vi "SelectMenu3.vi"(6 "Click Type":T1, 7 "Id":string, 8 "Point":T8, 9 "Item Index":u32, 10 "XRef":refnum<vi>, 11 "State In":T2={"Input Type"=variant(dbl 0.0), "Width"=0, "Typedef Name"="", "Value Type"=variant, "Selection"=0, "Options"=[], "Selections"=[], "Display Selections"=[], "Element Names"=[], "Typedef Name Width"=0, "Display Selection Width"=[], "Code Generated"=FALSE}) -> (0 "Reply":string[](array[string]), 3 "State Out":T2={"Input Type"=variant(dbl 0.0), "Width"=0, "Typedef Name"="", "Value Type"=variant, "Selection"=0, "Options"=[], "Selections"=[], "Display Selections"=[], "Element Names"=[], "Typedef Name Width"=0, "Display Selection Width"=[], "Code Generated"=FALSE})   [LabVIEW 2015, in "Read-Write-Signals.xnode"]
doc: "This ability VI is called after the user selects an item from a portion of the menu defined during BuildMenu. Click Type is the type of click that led to the building of the menu whose selection is being handled by this VI. ItemIndex is the index of the element in the array used when you specified the popup menu. Id is the id you associated with the item in BuildMenu3. Point is the location where the user clicked to build the menu relative to the top-left corner of the XNode. You can display a dialog in response to a user selection if you wish. Use Reply to inform LabVIEW of any actions it needs to take.\n\nDefault behavior: None.\n\nThis ability provides UI and OS messages are handled.\n\nSee also: BuildMenu3"
uses:
  Read-Write-Signals.xnode
  State.ctl
  Read-Write-Signals Item.ctl
  Read-Write-Signals Sub Item.ctl
  Read-Write-Signals Sub Item Type.ctl
  Read-Write-Signals Selection.ctl
  Read-Write-Signals Display Selection.ctl
  <vilib>/XNodeSupport/XNodePoint.ctl
  <vilib>/XNodeSupport/XNodeInt.ctl
  <vilib>/XNodeSupport/XNodeClickTypes.ctl
  <vilib>/regexp/Match Regular Expression.xnode
  <vilib>/XNodeSupport/NI_XNodeSupport.lvlib
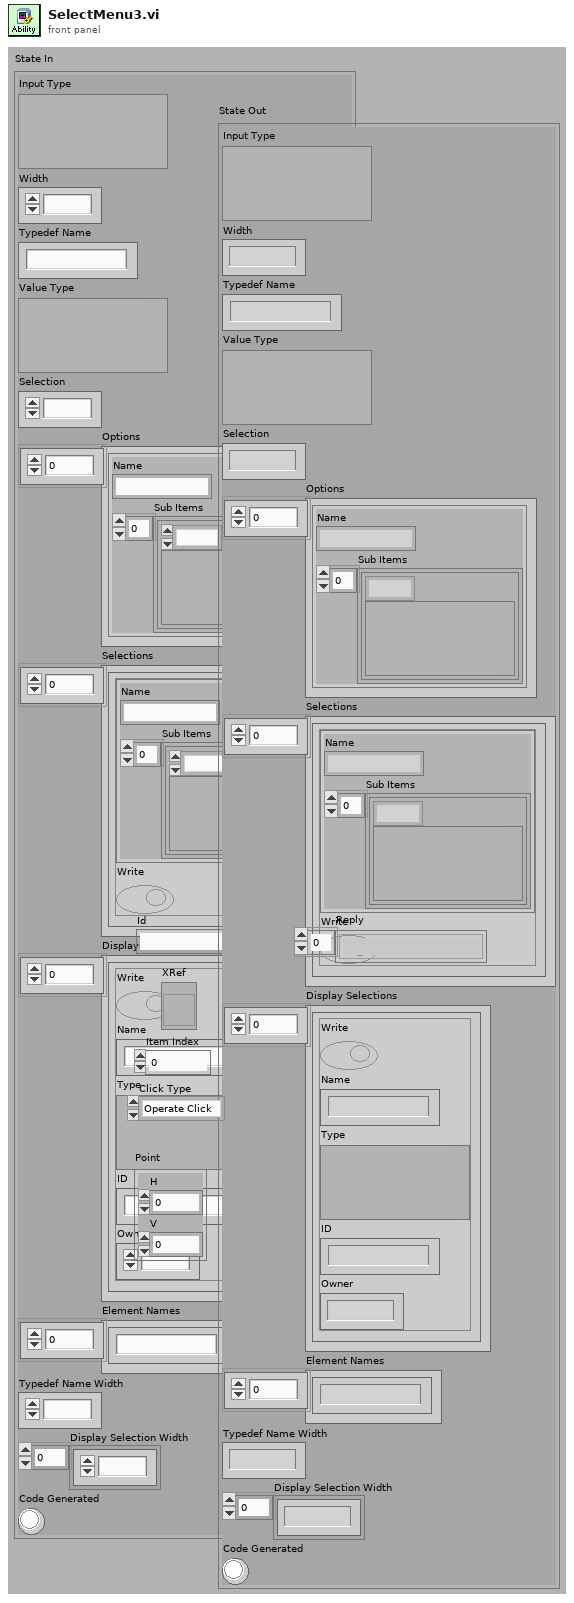
[diagram p1: front panel]
types:
  T1 = typedef "NI_XNodeSupport.lvlib/XNodeClickTypes.ctl" = enum32{"Operate Click", "Popup Click"}
  T2 = typedef "Read-Write-Signals.xnode/State.ctl" = cluster{"Input Type":variant, "Width":i32, "Typedef Name":string, "Value Type":variant, "Selection":i32, "Options":T3[], "Selections":T6[], "Display Selections":T7[], "Element Names":string[], "Typedef Name Width":i32, "Display Selection Width":i32[], "Code Generated":bool}
  T3 = typedef "Read-Write-Signals Item.ctl" = cluster{"Name":string, "Sub Items":T4[]}
  T4 = typedef "Read-Write-Signals Sub Item.ctl" = cluster{"Type":T5, "Value":variant}
  T5 = typedef "Read-Write-Signals Sub Item Type.ctl" = enum8{"Cluster Element", "Array Element", "Subarray"}
  T6 = typedef "Read-Write-Signals Selection.ctl" = cluster{"Item":T3, "Write":bool}
  T7 = typedef "Read-Write-Signals Display Selection.ctl" = cluster{"Write":bool, "Name":string, "Type":variant, "ID":string, "Owner":i32}
  T8 = typedef "NI_XNodeSupport.lvlib/XNodePoint.ctl" = cluster{"H":T9, "V":T9}
  T9 = typedef "NI_XNodeSupport.lvlib/XNodeInt.ctl" = i32
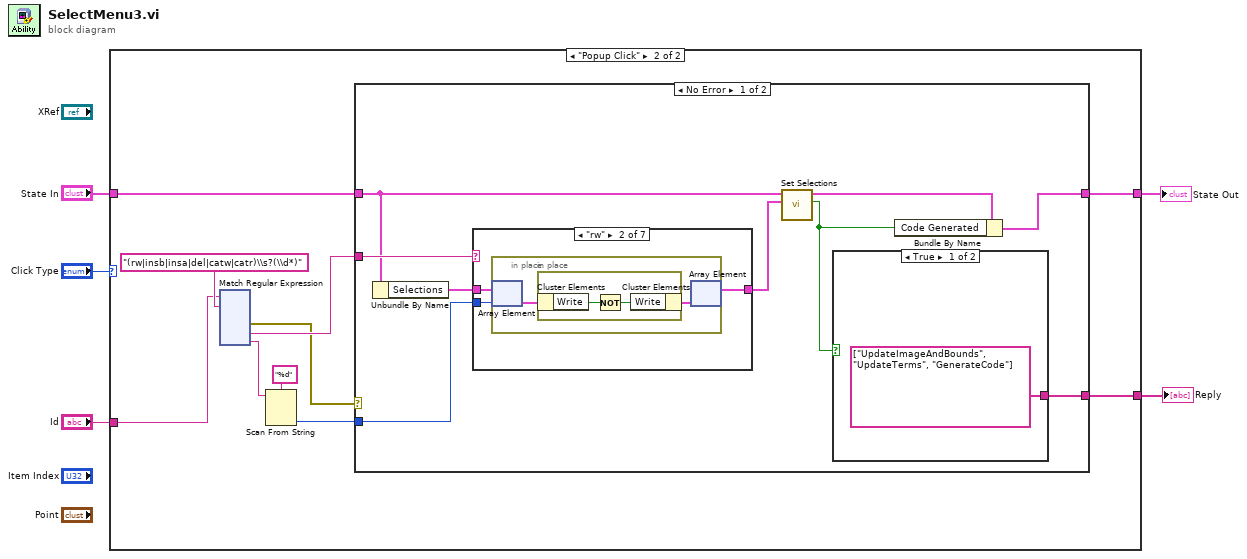
[diagram p0: block diagram]
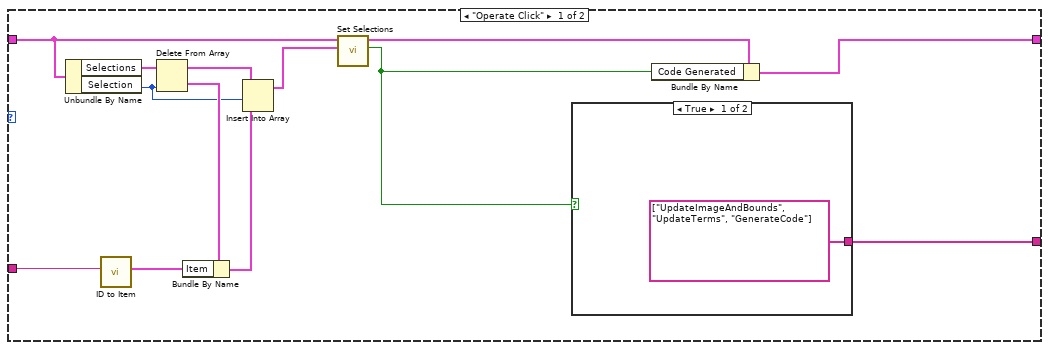
[diagram p2: hidden frame]
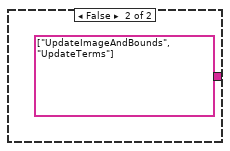
[diagram p3: hidden frame]
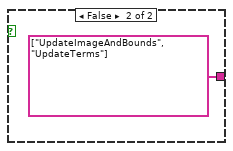
[diagram p4: hidden frame]
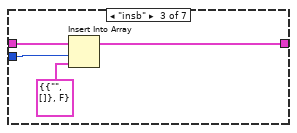
[diagram p6: hidden frame]
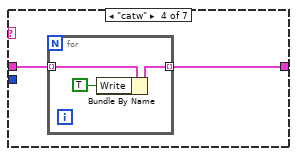
[diagram p7: hidden frame]
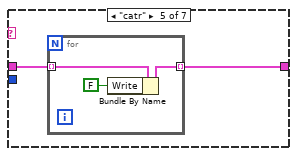
[diagram p8: hidden frame]
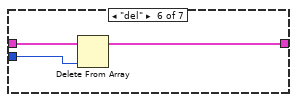
[diagram p9: hidden frame]
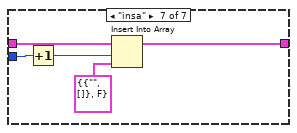
[diagram p10: hidden frame]
diagram:
  n1 = case shown="\"Popup Click\"" "Click Type" {
    tunnel: [w7 w28] -> w1
    tunnel: "State In" -> [w12 w29]
    tunnel: "Id" -> [w10 w23]
    tunnel: [w14 w26] -> w2
    frame "Operate Click" {
      n2 = Unbundle By Name(w12) -> ("Selections"=w18:T6[], "Selection"=w13:i32)
      n3 = call "ID to Item.vi"("ID"=w10) -> ("Item"=w9:T3)  [unwired: 10 in]
      n4 = Delete From Array(array=w18, index=w13) -> (deleted portion=w17:T6, array with subset deleted=w16:T6[])  [unwired: 1 in]
      n5 = Bundle By Name(cluster=w17, "Item"=w9) -> (w15:T6)
      n6 = Insert Into Array(array=w16, index=w13, new element=w15) -> (w11:T6[])
      n7 = call "Set Selections.vi"("Selections"=w11, "State in"=w12) -> ("All Valid"=w6:bool, "State out"=w8:T2)  [unwired: 8 in]
      n8 = case shown="True" w6 {
        tunnel: [string[] ["UpdateImageAndBounds", "UpdateTerms", "GenerateCode"] ("Reply") string[] ["UpdateImageAndBounds", "UpdateTerms"] ("Reply")] -> w14
        frame True {
        }
        frame False {
        }
      }
      n9 = Bundle By Name(cluster=w8, "Code Generated"=w6) -> (w7:T2)
    }
    frame "Popup Click" {
      n10 = xnode "Match Regular Expression"("input string"=w23, "regular expression"="(rw|insb|insa|del|catw|catr)\\s?(\\d*)") -> ("error out"=w21:errorcluster, "submatch 1"=w22:string, "submatch 2"=w24:string)  [unwired: 4 in, 4 out]
      n11 = Scan From String(format string="%d", input string=w24) -> (output 1=w27:i32)  [unwired: 3 in, 3 out]
      n12 = case shown="No Error" w21 {
        tunnel: w29 -> [w152 w189]
        tunnel: [w149 w189] -> w28
        tunnel: w27 -> [w156 _]
        tunnel: [w153 _] -> w26
        tunnel: w22 -> [w155 _]
        frame No Error {
          n13 = Unbundle By Name(w152) -> ("Selections"=w154:T6[])
          n14 = case shown="\"rw\"" w155 {
            tunnel: w154 -> [w159 w162 w170 w172 w177 w183 w188]
            tunnel: w156 -> [_ w161 w169 _ _ w181 w187]
            tunnel: [w159 w160 w168 w171 w176 w182 w186] -> w151
            frame Default {
            }
            frame "rw" {
              n15 = in-place {
                n16 = in-place-array #1(w162, w161) -> (w164:T6)
                n17 = in-place {
                  n18 = in-place-cluster #2(w164) -> ("Write"=w166:bool)
                  n19 = Not(x=w166) -> (.not. x?=w165:bool)
                  n20 = in-place-cluster #2("Write"=w165) -> (w163:T6)
                }
                n21 = in-place-array #1(w163) -> (w160:T6[])  [unwired: 1 out]
              }
            }
            frame "insb" {
              n22 = Insert Into Array(array=w170, index=w169, new element=T6 {"Item"={"Name"="", "Sub Items"=[]}, "Write"=FALSE} ("new element/subarray")) -> (w168:T6[])
            }
            frame "catw" {
              n23 = for {
                tunnel: w172 -> [w175] mode=indexing
                tunnel: [w173] -> w171 mode=indexing
                n24 = Bundle By Name(cluster=w175, "Write"=TRUE) -> (w173:T6)
              }
            }
            frame "catr" {
              n25 = for {
                tunnel: w177 -> [w180] mode=indexing
                tunnel: [w178] -> w176 mode=indexing
                n26 = Bundle By Name(cluster=w180, "Write"=FALSE) -> (w178:T6)
              }
            }
            frame "del" {
              n27 = Delete From Array(array=w183, index=w181) -> (array with subset deleted=w182:T6[])  [unwired: 1 in, 1 out]
            }
            frame "insa" {
              n28 = Increment(x=w187) -> (x+1=w185:i32)
              n29 = Insert Into Array(array=w188, index=w185, new element=T6 {"Item"={"Name"="", "Sub Items"=[]}, "Write"=FALSE} ("new element/subarray")) -> (w186:T6[])
            }
          }
          n30 = call "Set Selections.vi"("Selections"=w151, "State in"=w152) -> ("All Valid"=w148:bool, "State out"=w150:T2)  [unwired: 8 in]
          n31 = case shown="True" w148 {
            tunnel: [string[] ["UpdateImageAndBounds", "UpdateTerms", "GenerateCode"] ("Reply") string[] ["UpdateImageAndBounds", "UpdateTerms"] ("Reply")] -> w153
            frame True {
            }
            frame False {
            }
          }
          n32 = Bundle By Name(cluster=w150, "Code Generated"=w148) -> (w149:T2)
        }
        frame Error {
        }
      }
    }
  }
  "State Out" <- w1
  "Reply" <- w2
